vi "CAN react.vi"(7 "Time Stamp":timestamp format="%<%x %.3X>T", 8 "error in":errorcluster, 9 "Data":u8[](array[numeric]), 10 "COB-ID":u32, 11 "CANopen in":refnum<class "CANopen.lvclass">) -> (0 "error out":errorcluster, 3 "CANopen out":refnum<class "CANopen.lvclass">)   [LabVIEW 2026, in "canopen_.lvlib" / "CANopen.lvclass"]
doc: "Starts the task that reads messages and tries to handle them."
uses:
  CANopen.lvclass
  CANopen.lvclass/CANopen.ctl
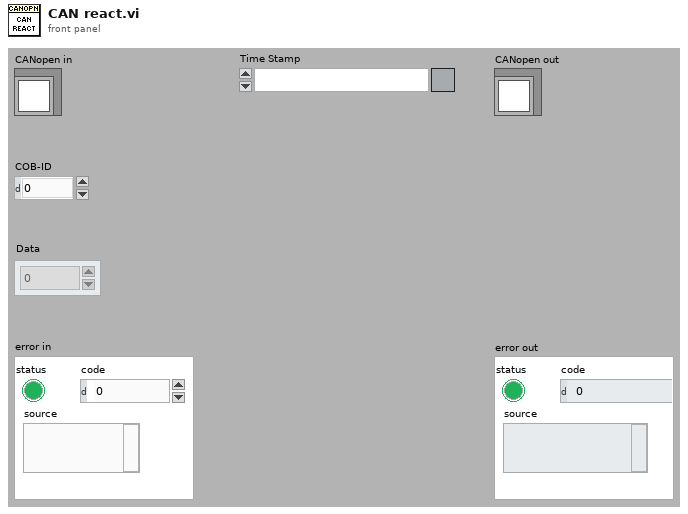
[diagram p1: front panel]
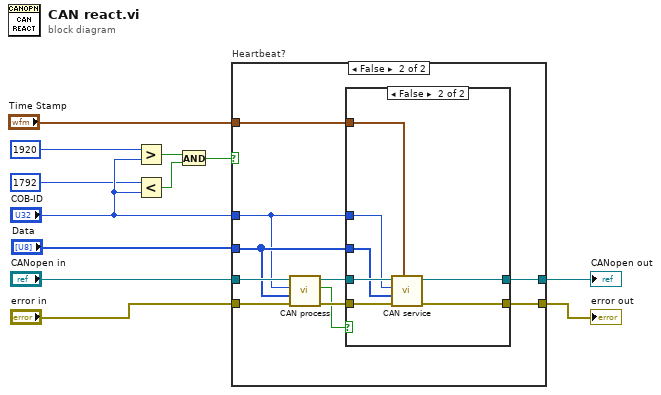
[diagram p0: block diagram]
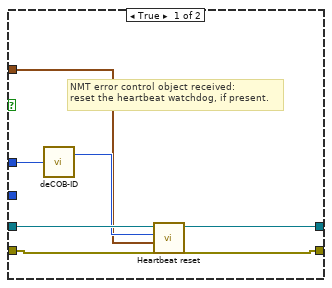
[diagram p2: hidden frame]
diagram:
  n1 = Greater?(x=u32 1920, y="COB-ID") -> (0:w5:bool)
  n2 = Less?(x=u32 1792, y="COB-ID") -> (x < y?=w4:bool)
  n3 = And(x=w5, y=w4) -> (x .and. y?=w3:bool)
  n4 = case "Heartbeat?" shown="False" w3 {
    tunnel: "CANopen in" -> [w17 w25]
    tunnel: "error in" -> [w14 w24]
    tunnel: "Data" -> [_ w23]
    tunnel: [w16 w22] -> w10
    tunnel: [w14 w21] -> w9
    tunnel: "COB-ID" -> [w18 w20]
    tunnel: "Time Stamp" -> [w13 w19]
    frame True {
      # "NMT error control object received:\nreset the heartbeat watchdog, if present."
      n5 = call "deCOB-ID.vi"("Cob ID"=w18) -> ("Node ID"=w15:u8)  [unwired: 1 out]
      n6 = call "Heartbeat reset.vi"("New Beat"=w13, "Node ID"=w15, "CANopen in"=w17) -> ("CANopen out"=w16:refnum<class "CANopen.lvclass">)  [unwired: 8 in]
    }
    frame False {
      n7 = call "CAN process.vi"("error in (no error)"=w24, "Data"=w23, "COB id"=w20, "CANopen in"=w25) -> ("error out"=w28:errorcluster, "Processed?"=w27:bool, "CANopen out"=w26:refnum<class "CANopen.lvclass">)  [unwired: 1 out]
      n8 = case shown="False" w27 {
        tunnel: w28 -> [w30 w37]
        tunnel: [w30 w36] -> w21
        tunnel: [w29 w35] -> w22
        tunnel: w26 -> [w29 w34]
        tunnel: w20 -> [_ w33]
        tunnel: w23 -> [_ w32]
        tunnel: w19 -> [_ w31]
        frame True {
        }
        frame False {
          n9 = call "CAN service.vi"("Time Stamp"=w31, "error in"=w37, "Data"=w32, "COB-ID"=w33, "CANopen in"=w34) -> ("error out"=w36:errorcluster, "CANopen out"=w35:refnum<class "CANopen.lvclass">)  [unwired: 5 in]
        }
      }
    }
  }
  "CANopen out" <- w10
  "error out" <- w9
